vi "DiscreteHysInv.vi"(1 "En H Inv":bool, 2 "DBO Para":T1, 3 "input Yi":dbl[](array[numeric])=[0.0, 0.0, 0.0]) -> (0 "Xi":dbl[](array[numeric]))   [LabVIEW 2011]
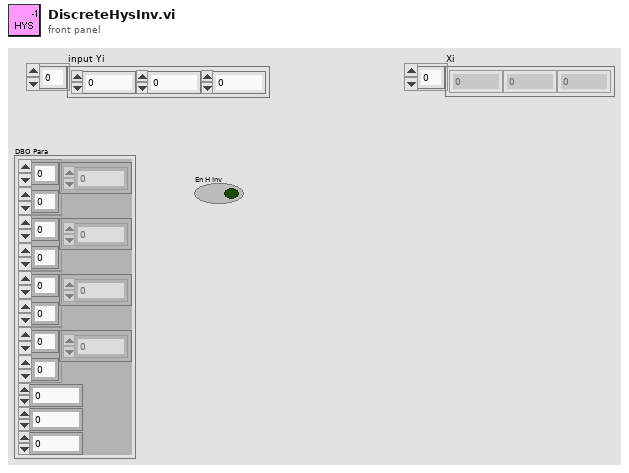
[diagram p1: front panel]
types:
  T1 = cluster{dbl[][], dbl[][], dbl[][], dbl[][], dbl, dbl, dbl}
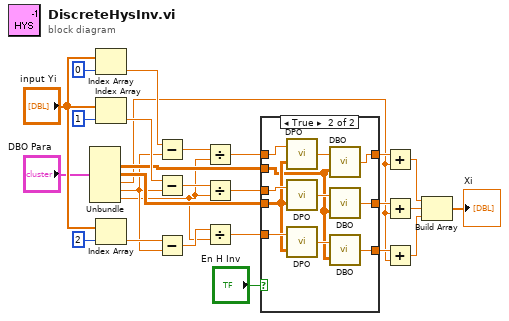
[diagram p0: block diagram]
diagram:
  n1 = Unbundle("DBO Para") -> (w4:dbl[][], w5:dbl[][], w3:dbl, w2:dbl, w1:dbl)  [unwired: 2 out]
  n2 = Index Array(array="input Yi", index=0) -> (element=w21:dbl)
  n3 = Index Array(array="input Yi", index=1) -> (element=w20:dbl)
  n4 = Index Array(array="input Yi", index=2) -> (element=w19:dbl)
  n5 = Subtract(x=w21, y=w2) -> (x-y=w14:dbl)
  n6 = Subtract(x=w20, y=w2) -> (x-y=w16:dbl)
  n7 = Subtract(x=w19, y=w2) -> (x-y=w15:dbl)
  n8 = Divide(x=w14, y=w1) -> (x/y=w13:dbl)
  n9 = Divide(x=w16, y=w1) -> (x/y=w12:dbl)
  n10 = Divide(x=w15, y=w1) -> (x/y=w11:dbl)
  n11 = case shown="True" "En H Inv" {
    tunnel: w13 -> [w30 w41]
    tunnel: w12 -> [w29 w40]
    tunnel: w11 -> [w28 w39]
    tunnel: [w30 w38] -> w10
    tunnel: [w29 w35] -> w9
    tunnel: [w28 w33] -> w8
    tunnel: w5 -> [_ w32]
    tunnel: w4 -> [_ w31]
    frame False {
    }
    frame True {
      n12 = call "DPO.vi"("S"=w32, "x"=w41) -> ("y"=w37:dbl)
      n13 = call "DPO.vi"("S"=w32, "x"=w40) -> ("y"=w36:dbl)
      n14 = call "DPO.vi"("S"=w32, "x"=w39) -> ("y"=w34:dbl)
      n15 = call "DBO.vi"("H"=w31, "x"=w37) -> ("y"=w38:dbl)
      n16 = call "DBO.vi"("H"=w31, "x"=w36) -> ("y"=w35:dbl)
      n17 = call "DBO.vi"("H"=w31, "x"=w34) -> ("y"=w33:dbl)
    }
  }
  n18 = Add(x=w10, y=w3) -> (x+y=w22:dbl)
  n19 = Add(x=w9, y=w3) -> (x+y=w17:dbl)
  n20 = Add(x=w8, y=w3) -> (x+y=w18:dbl)
  n21 = Build Array(w22, w17, w18) -> (→"Xi":dbl[])
